vi "GetSystemPath.vi"(4 "编译状态":enum16{"代码版", "打包版"}(ring)) -> (1 "Relative path":path)   [LabVIEW 2018]
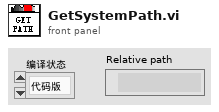
[diagram p1: front panel]
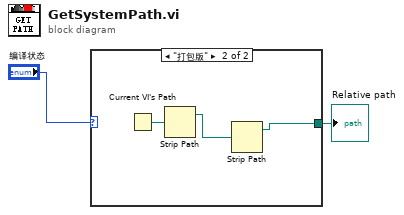
[diagram p0: block diagram]
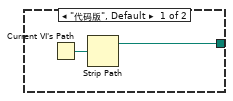
[diagram p2: hidden frame]
diagram:
  n1 = case shown="\"打包版\"" "编译状态" {
    tunnel: [w3 w5] -> w1
    frame "代码版", Default {
      n2 = Current VI's Path() -> (path=w4:path)
      n3 = Strip Path(path=w4) -> (stripped path=w3:path)  [unwired: 1 out]
    }
    frame "打包版" {
      n4 = Current VI's Path() -> (path=w7:path)
      n5 = Strip Path(path=w7) -> (stripped path=w6:path)  [unwired: 1 out]
      n6 = Strip Path(path=w6) -> (stripped path=w5:path)  [unwired: 1 out]
    }
  }
  "Relative path" <- w1
